vi "RunTest.vi"(8 "error in (no error)":errorcluster, 11 "Prueba05 in":refnum<class "Prueba05.lvclass">) -> (0 "error out":errorcluster, 2 "resultado":string, 3 "Prueba05 out":refnum<class "Prueba05.lvclass">)   [LabVIEW 2019, in "Prueba05.lvclass"]
uses:
  Prueba05.lvclass
  Prueba04/Control/Slide.ctl
  Prueba05.lvclass/Prueba05.ctl
  ClusterGEN.ctl
  <vilib>/Utility/miscctls.llb/LVRowAndColumnTypeDef.ctl
  <vilib>/Utility/error.llb/DialogType.ctl
  QMH/Message Queue/Enqueue Message (Single).vi
  <vilib>/Utility/error.llb/Error Cluster From Error Code.vi
  <vilib>/ErrorRing/Error Ring.xnode
  Prueba/Prueba.lvclass
  Prueba04/Prueba04.lvclass
  QMH/User Event - Stop/User Event - Stop.lvlib
  QMH/Message Queue/Message Queue.lvlib
panel:
  out "cumple_no_cumple":bool
  in  "Tab":enum32{"Page 1", "Page 2"}(tab)
  in  "generar_1":bool
  out "frecuencia":dbl
  in  "seguir":bool
  out "voltaje1":dbl format="%.1f"
  out "frecuencia1":dbl format="%.1f"
  in  "AjusteAmp":T1=50.0 caption="Ajuste de amplitud [mV]" scale=0.0..500.0
  in  "guardar":bool
  out "Pict Ring 2":u16(ring)
  out "Pict Ring":u16(ring)
  out "voltajeGuardado":dbl format="%.1f"
  in  "Tabla_A":string[][](table)
  out "voltaje2":dbl format="%.1f"
  out "frecuencia2":dbl format="%.1f"
  out "no_cumple":bool
  out "cumple":bool
  in  "generar_2":bool
  out "frecuencia2":dbl format="%.1f"
  in  "salir":bool
  # "Generación Señal de Prueba"
  # "Hz"
  # "Frecuencia"
  # "5. Ponderaciones frecuenciales y temporales a 1 KHz. IEC 61672-3: 2006 Cláusula 13"
  # "Monitoreo"
  # "Frecuencia"
  # "Hz"
  # "Voltaje"
  # "mV"
  # "Hz"
  # "mV"
  # "Cumple"
  # "No Cumple"
  # "Monitoreo"
  # "Frecuencia"
  # "Hz"
  # "Voltaje"
  # "mV"
  # "Voltaje"
  # "Frecuencia"
  # "5. Ponderaciones frecuenciales y temporales a 1 KHz. IEC 61672-3: 2006 Cláusula 13"
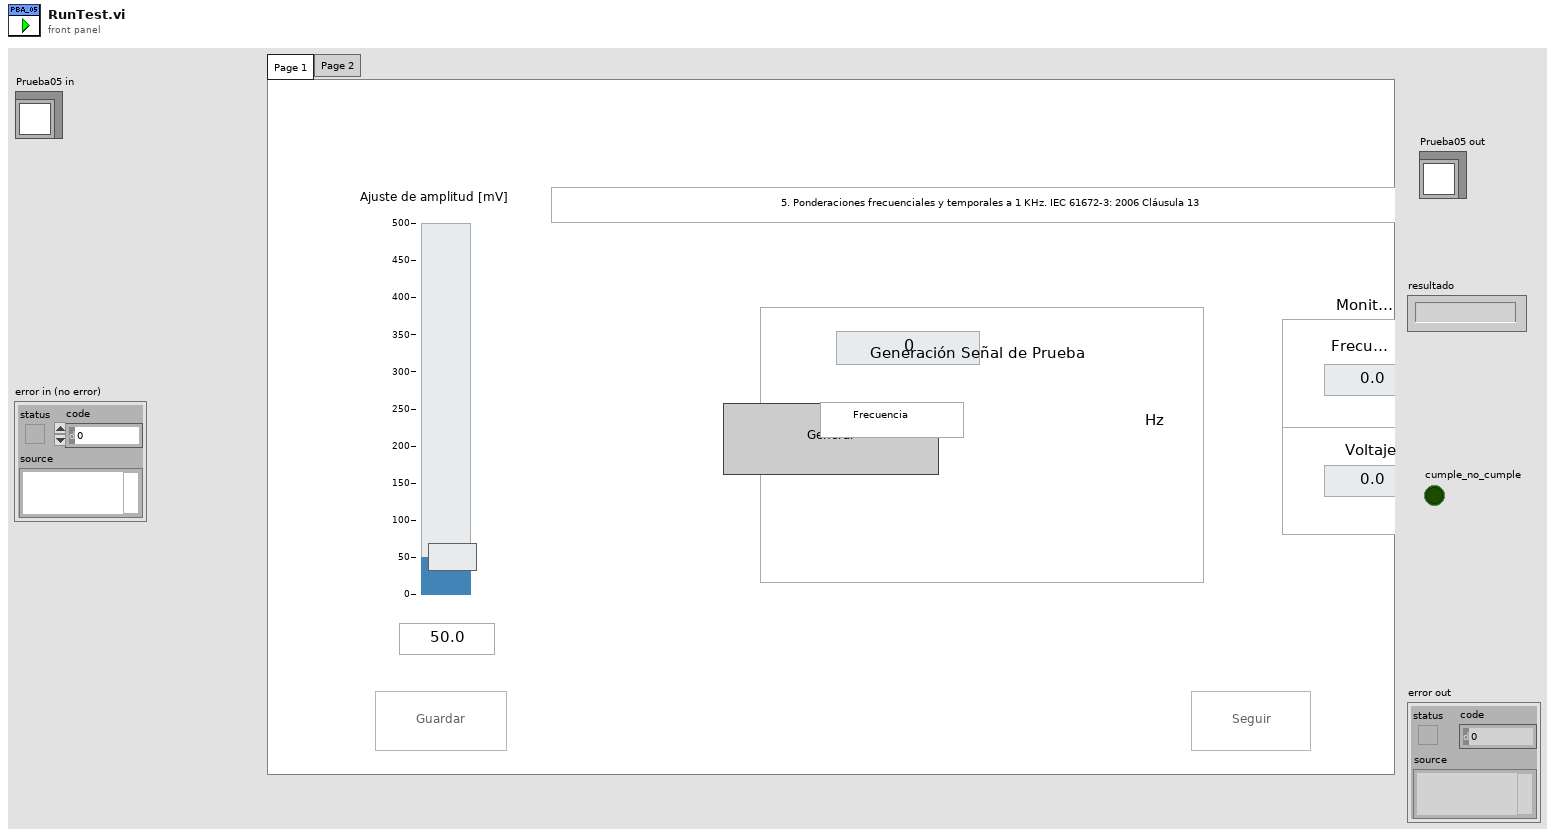
[diagram p1: front panel]
types:
  T1 = typedef "Prueba04.lvclass/Slide.ctl" = dbl
  T2 = typedef "Message Queue.lvlib/All Message Queues.ctl" = cluster{"MHL":refnum<queue>, "Inst_CNT90":refnum<queue>, "Inst_DS360":refnum<queue>, "Inst_Keithley2002":refnum<queue>, "Inst_DAQ":refnum<queue>, "BD":refnum<queue>, "Pistofono":refnum<queue>, "Nexus":refnum<queue>}
  T3 = enum8{"Enabled", "Disabled", "Disabled and Grayed Out"}
  T4 = typedef "LVRowAndColumnTypeDef.ctl" = cluster{"Row":i32, "Column":i32}
  T5 = enum32{"Page 1", "Page 2", "Page 3", "Page 4", "Page 5", "Page 6", "Page 7"}
  T6 = typedef "Prueba05.lvclass/ClusterGEN.ctl" = cluster{"frec":dbl, "amp":dbl}
  T7 = cluster{"ControlName":string, "ControlReference":refnum<vi>}[]
  T8 = typedef "DialogType.ctl" = u16
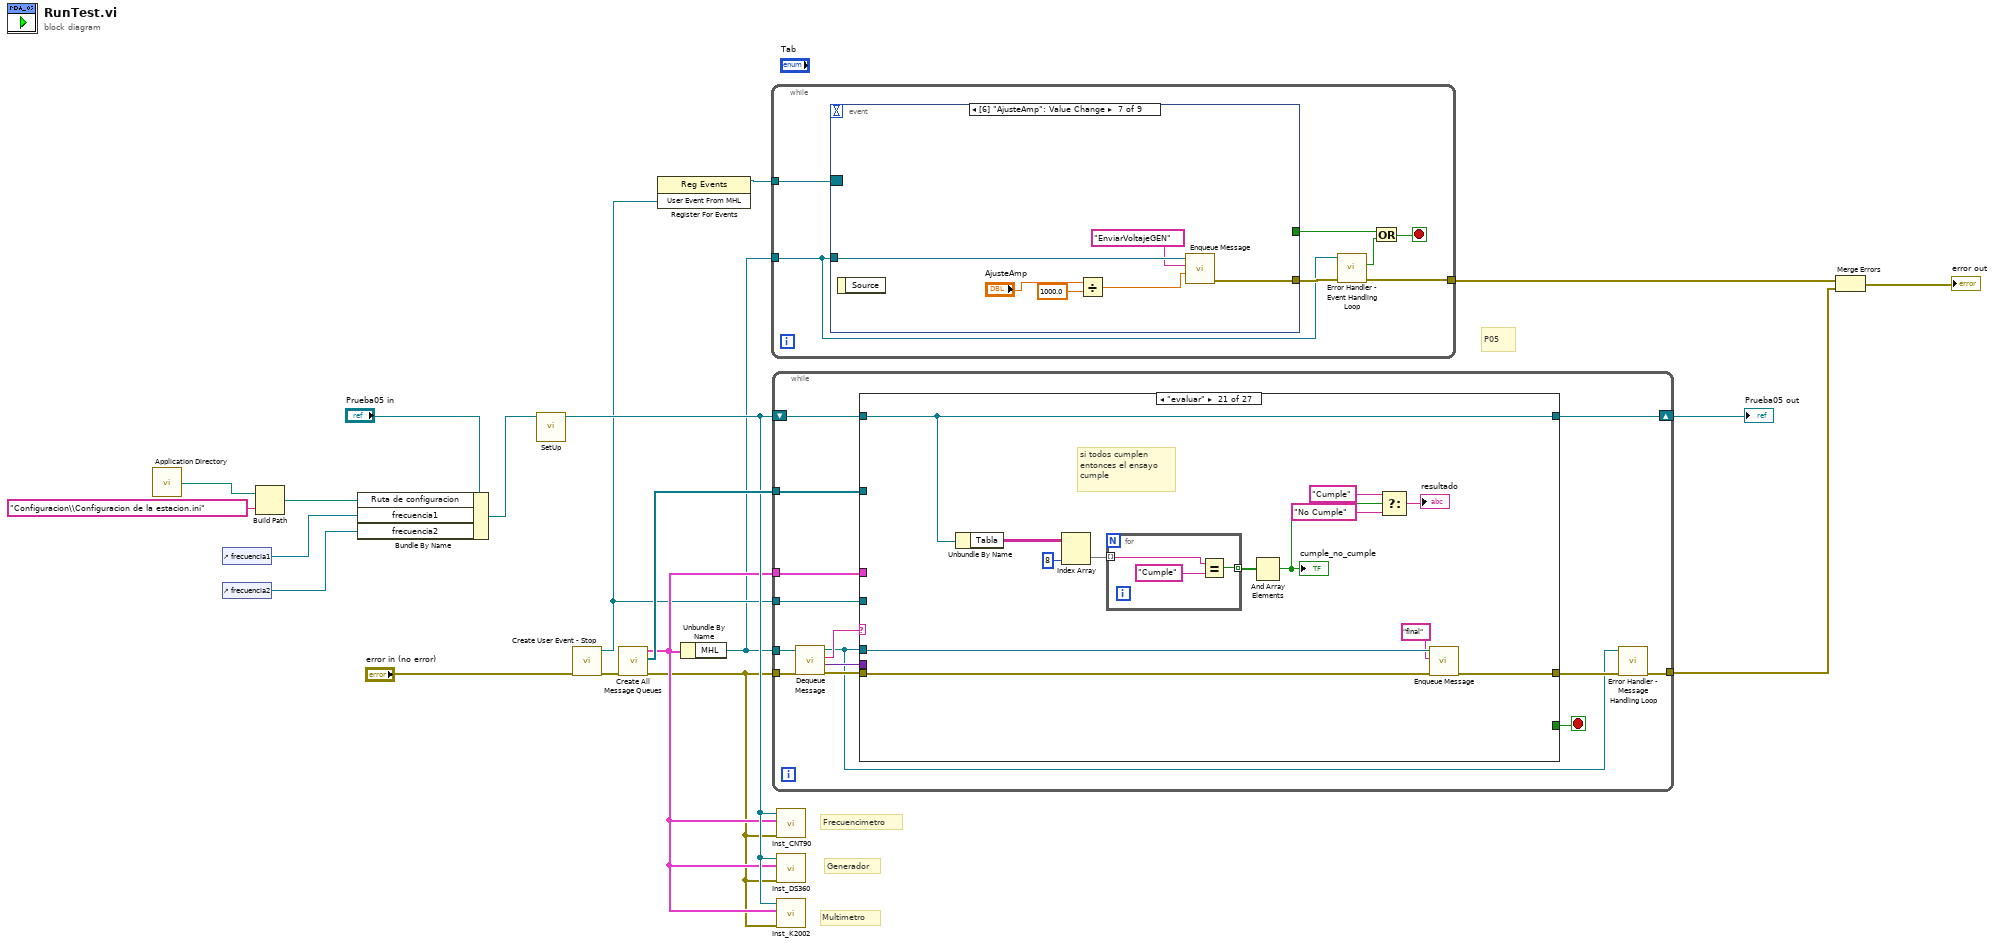
[diagram p0: block diagram]
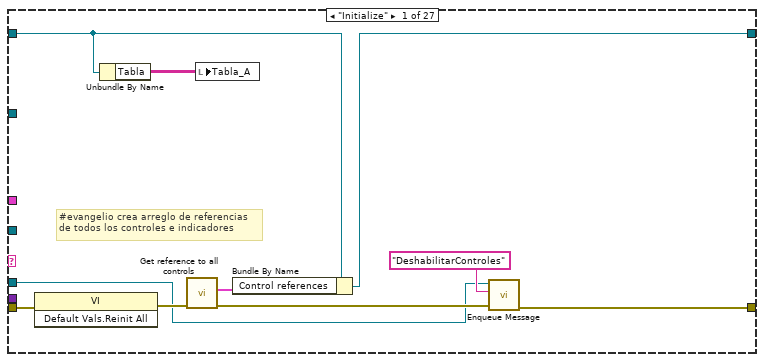
[diagram p2: hidden frame]
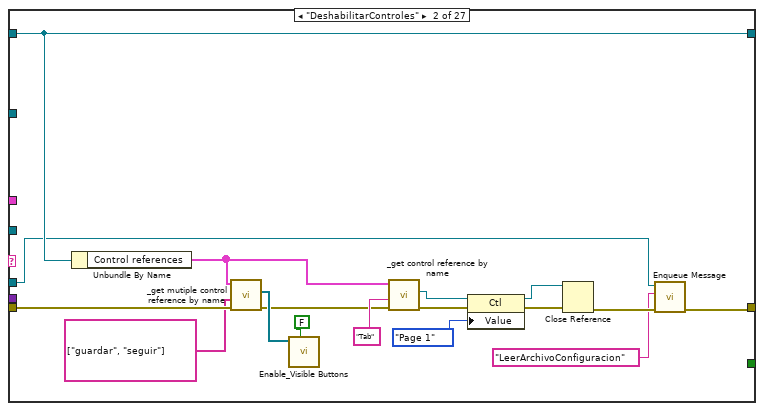
[diagram p3: hidden frame]
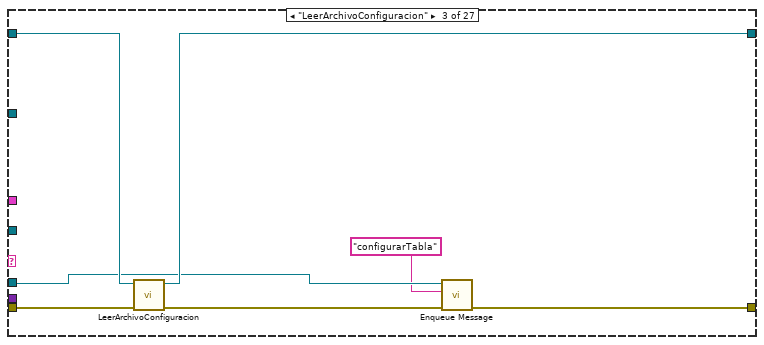
[diagram p4: hidden frame]
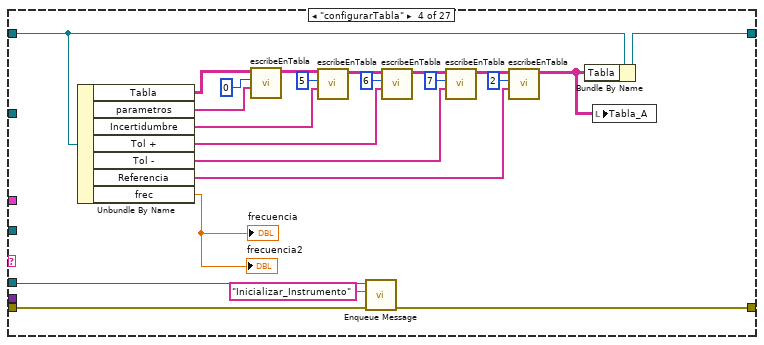
[diagram p5: hidden frame]
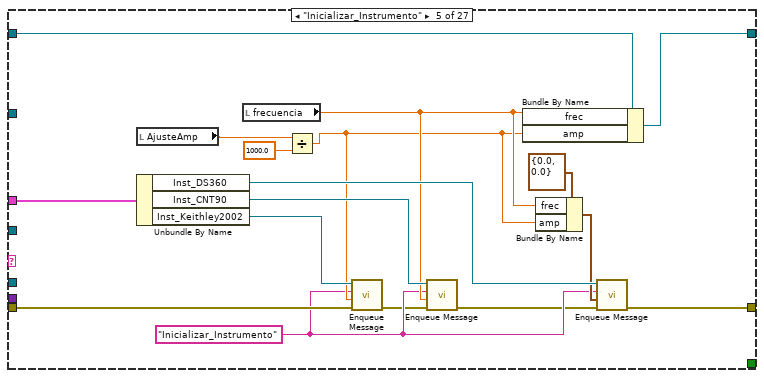
[diagram p6: hidden frame]
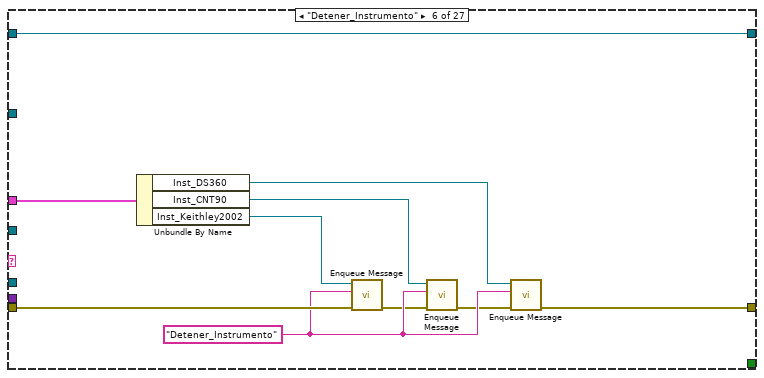
[diagram p7: hidden frame]
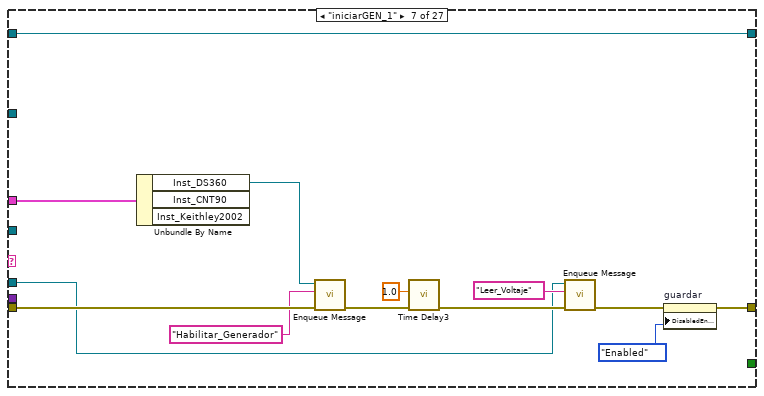
[diagram p8: hidden frame]
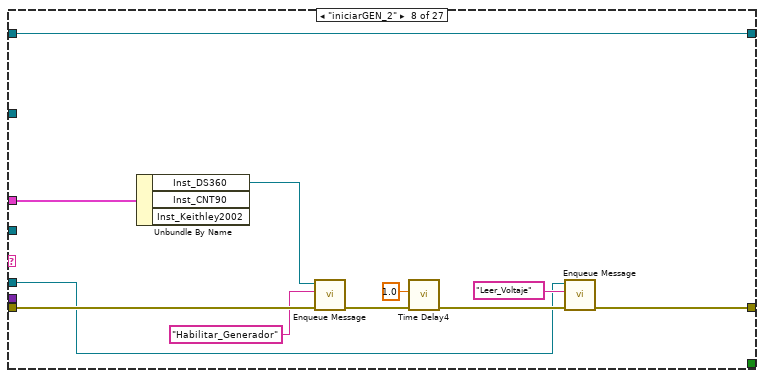
[diagram p9: hidden frame]
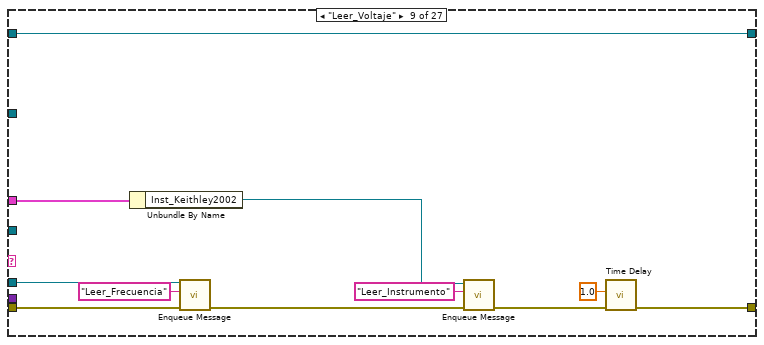
[diagram p10: hidden frame]
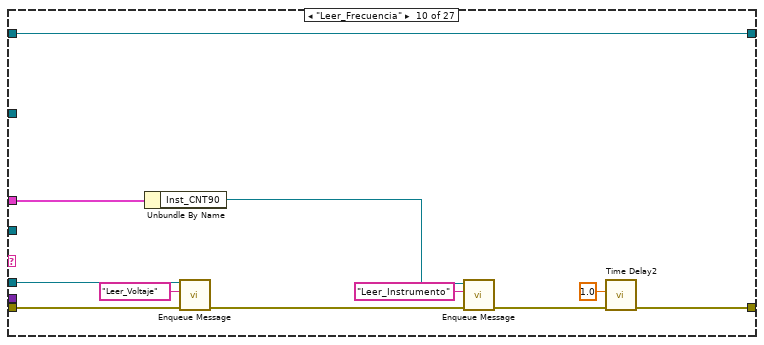
[diagram p11: hidden frame]
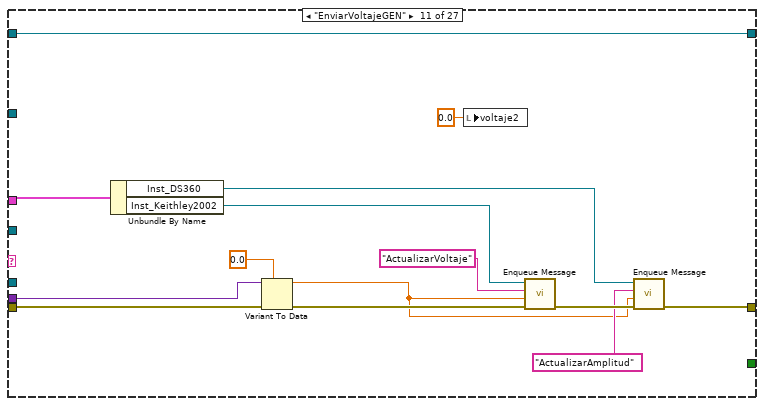
[diagram p12: hidden frame]
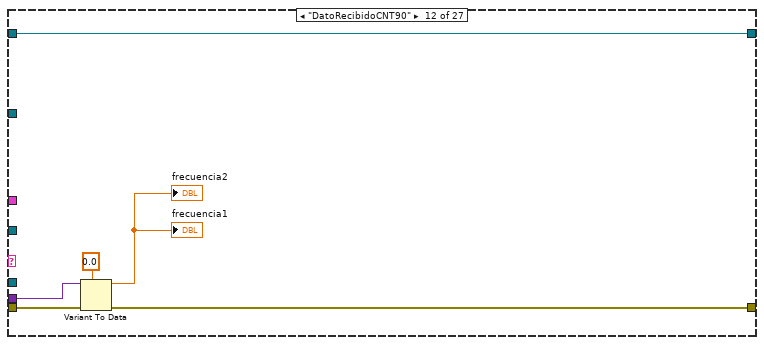
[diagram p13: hidden frame]
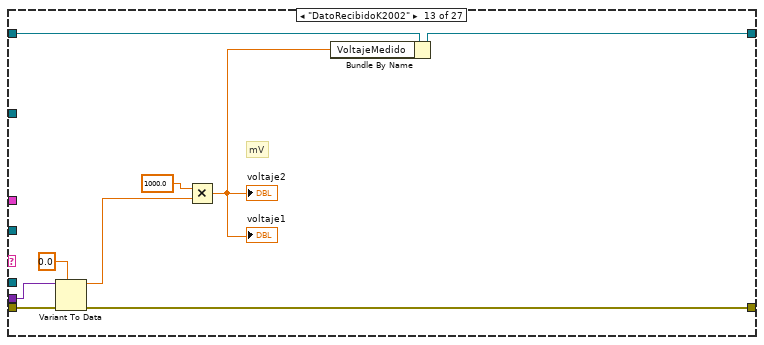
[diagram p14: hidden frame]
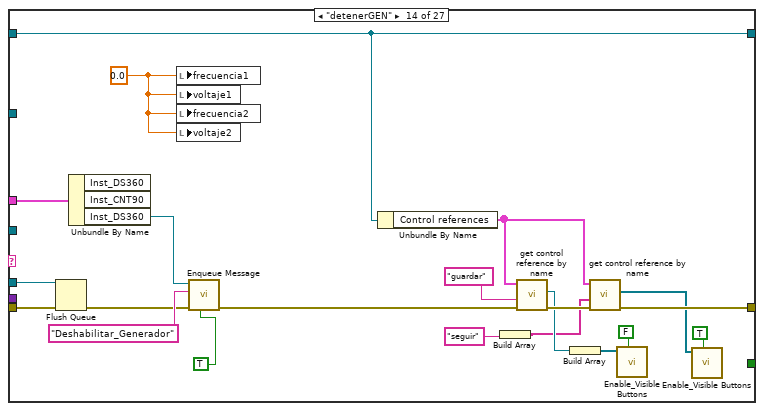
[diagram p15: hidden frame]
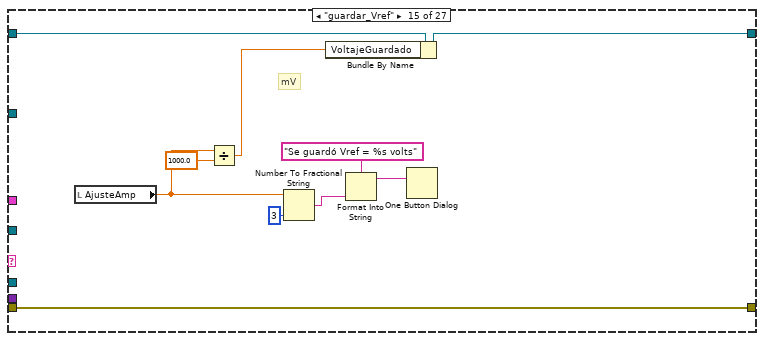
[diagram p16: hidden frame]
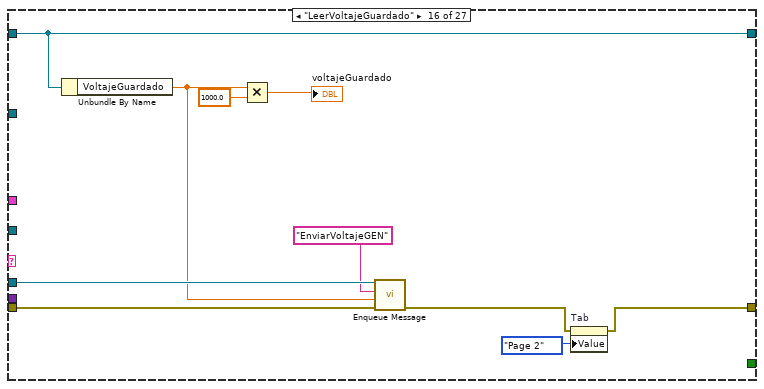
[diagram p17: hidden frame]
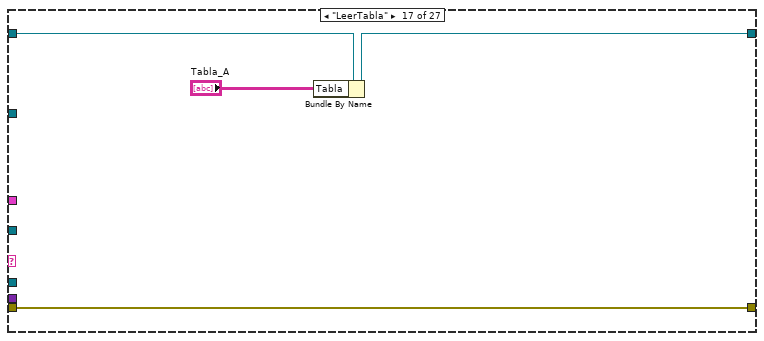
[diagram p18: hidden frame]
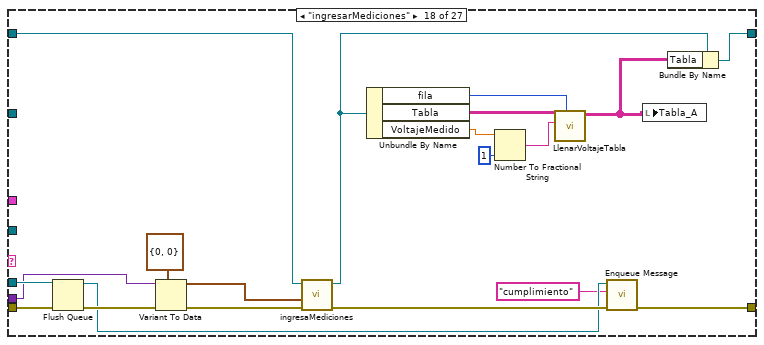
[diagram p19: hidden frame]
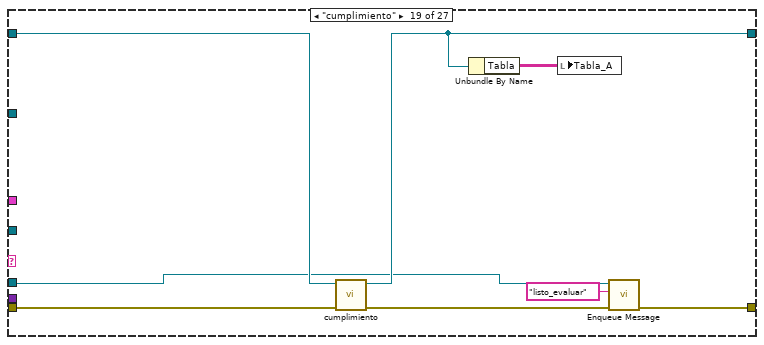
[diagram p20: hidden frame]
diagram:
  # "P05"
  # "Multimetro"
  # "Generador"
  # "Frecuencimetro"
  n1 = call <vilib>:"Application Directory.vi"() -> ("Application Directory"=w15:path)
  n2 = control-ref of="frecuencia1"() -> (w2:refnum<vi>)
  n3 = control-ref of="frecuencia2"() -> (w1:refnum<vi>)
  n4 = Build Path(base path=w15, name or relative path="Configuracion\\Configuracion de la estacion.ini") -> (appended path=w14:path)
  n5 = Bundle By Name(cluster="Prueba05 in", "Ruta de configuracion"=w14, "frecuencia1"=w2, "frecuencia2"=w1) -> (w12:refnum<class "Prueba05.lvclass">)
  n6 = call-dynamic "SetUp.vi"("Prueba05 in"=w12) -> ("Prueba05 out"=w7:refnum<class "Prueba05.lvclass">)  [unwired: 9 in, 1 out]
  n7 = call "Create User Event - Stop.vi"("error in (no error)"="error in (no error)") -> ("error out"=w11:errorcluster, "User Event From MHL"=w4:refnum<user-event>)  [unwired: 9 in]
  n8 = call "Create All Message Queues.vi"("error in (no error)"=w11) -> ("error out"=w5:errorcluster, "PL Queues Array"=w9:refnum<queue>[], "All Message Queues out"=w6:T2)  [unwired: 8 in]
  n9 = register-events(w4) -> (reference out=w8:refnum<event-registration>)  [unwired: 2 in, 1 out]
  n10 = Unbundle By Name(w6) -> ("MHL"=w3:refnum<queue>)
  n11 = while {
    tunnel: [w24] -> w20
    tunnel: w8 -> [w26]
    tunnel: w3 -> [w21]
    stop <- w27 stop-if-true
    n12 = event shown="[6] \"AjusteAmp\": Value Change" {
      selector: w26 -> [_ _ _ _ _ _ _ _ _]
      dyn-events: _ -> [_ _ _ _ _ _ _ _ _]
      timeout: _ -> [_ _ _ _ _ _ _ _ _]
      tunnel: [w32 _ w39 w44 w55 w57 w66 w67 w78] -> w25
      tunnel: w21 -> [w30 _ w41 w49 w54 w59 w65 w71 w82]
      tunnel: [_ w33 _ _ _ _ _ _ _] -> w22
      event "salir": Value Change {
        n13 = event-data() -> ()  [unwired: 1 in, 1 out]
        n14 = call-poly "Enqueue Message.vi"("Message"="Detener_Instrumento", "Message Queue"=w30) -> ("dup Message Queue"=w29:refnum<queue>)  [unwired: 8 in, 1 out]
        n15 = call-poly "Enqueue Message.vi"("Message"="Exit", "Message Queue"=w29) -> ("error out"=w32:errorcluster)  [unwired: 8 in, 1 out]
      }
      event User Event {
        n16 = event-data() -> ("User Event"=w35:string, "Event Data"=w34:variant)  [unwired: 1 in]
        n17 = case shown="\"Exit EHL\"" w35 {
          tunnel: w34 -> [_ w37]
          tunnel: [_ w36] -> w33
          frame Default {
          }
          frame "Exit EHL" {
            # "#evangelio Termina\nla ejecucion del EHL"
            n18 = Variant To Data(type=TRUE, Variant=w37) -> (data=w36:bool)  [unwired: 1 in, 1 out]
          }
        }
      }
      event Panel Close? {
        w40 = TRUE
        n19 = event-data() -> ()  [unwired: 1 in, 1 out]
        n20 = call-poly "Enqueue Message.vi"("Priority Message? (F)"=w40, "Message"="Confirmar Salida", "Message Queue"=w41) -> ("error out"=w39:errorcluster)  [unwired: 7 in, 1 out]
        n21 = event-data("Discard?"=w40) -> ()  [unwired: 1 in, 1 out]
      }
      event "generar_1": Value Change {
        n22 = event-data() -> ("NewVal"=w48:bool)  [unwired: 1 in]
        n23 = Select(t="iniciarGEN_1" ("Message"), s=w48, f="detenerGEN" ("Message")) -> (s? t:f=w45:string)
        n24 = call-poly "Enqueue Message.vi"("Priority Message? (F)"=TRUE, "Message"=w45, "Message Queue"=w49) -> ("error out"=w44:errorcluster)  [unwired: 7 in, 1 out]
      }
      event "generar_2": Value Change {
        n25 = event-data() -> ("NewVal"=w53:bool)  [unwired: 1 in]
        n26 = Select(t="iniciarGEN_2", s=w53, f="detenerGEN") -> (s? t:f=w50:string)
        n27 = call-poly "Enqueue Message.vi"("Message"=w50, "Message Queue"=w54) -> ("error out"=w55:errorcluster)  [unwired: 8 in, 1 out]
      }
      event "seguir": Value Change {
        n28 = event-data() -> ()  [unwired: 1 in, 1 out]
        n29 = call-poly "Enqueue Message.vi"("Message"="LeerVoltajeGuardado", "Message Queue"=w59) -> ("error out"=w58:errorcluster)  [unwired: 8 in, 1 out]
        n30 = property on="Tab" class="TabCtl (strict)"(error in=w58, "Value"=enum32{"Page 1", "Page 2"}."Page 2" ("Tab")) -> (error out=w57:errorcluster)  [unwired: 1 in, 1 out]
      }
      event Value Change {
        n31 = event-data() -> ()  [unwired: 1 in, 1 out]
        n32 = Divide(x="AjusteAmp", y=T1 1000.0) -> (x/y=w61:T1)
        n33 = call-poly "Enqueue Message.vi"("Message Data"=w61, "Message"="EnviarVoltajeGEN", "Message Queue"=w65) -> ("error out"=w66:errorcluster)  [unwired: 7 in, 1 out]
      }
      event "guardar": Value Change {
        n34 = event-data() -> ()  [unwired: 1 in, 1 out]
        n35 = call-poly "Enqueue Message.vi"("Message"="guardar_Vref", "Message Queue"=w71) -> ("error out"=w68:errorcluster)  [unwired: 8 in, 1 out]
        n36 = property on="seguir" class="Bool"(error in=w68, "DisabledEnum"=T3."Enabled" ("Disabled")) -> (error out=w67:errorcluster)  [unwired: 1 in, 1 out]
      }
      event "Tabla_A": Value Change {
        n37 = event-data() -> ("CtlRef"=w81:refnum<vi>)  [unwired: 1 in]
        n38 = Flush Queue(queue=w82) -> (queue out=w74:refnum<queue>, error out=w72:errorcluster)  [unwired: 1 in, 1 out]
        n39 = property class="Tbl (strict)"(reference=w81, error in=w72) -> (error out=w73:errorcluster, "Selection Start"=w77:T4)  [unwired: 1 out]
        n40 = call-poly "Enqueue Message.vi"("error in (no error)"=w73, "Message"="LeerTabla", "Message Queue"=w74) -> ("error out"=w79:errorcluster, "dup Message Queue"=w80:refnum<queue>)  [unwired: 7 in]
        n41 = call-poly "Enqueue Message.vi"("error in (no error)"=w79, "Message Data"=w77, "Message"="ingresarMediciones", "Message Queue"=w80) -> ("error out"=w78:errorcluster)  [unwired: 6 in, 1 out]
      }
    }
    n42 = call "Error Handler - Event Handling Loop.vi"("error in (no error)"=w25, "Message Queue"=w21) -> ("dup error in"=w24:errorcluster, "Error?"=w23:bool)  [unwired: 7 in, 1 out]
    n43 = Or(x=w22, y=w23) -> (x .or. y?=w27:bool)
  }
  n44 = while {
    tunnel: [w87] -> w19
    shift-right: [w95] -> w17
    shift-left: w7 -> [w96]
    tunnel: w5 -> [w94]
    tunnel: w3 -> [w92]
    tunnel: w6 -> [w86]
    tunnel: w9 -> [w85]
    tunnel: w4 -> [w84]
    stop <- w83 stop-if-true
    n45 = call "Dequeue Message.vi"("error in (no error)"=w94, "Message Queue"=w92) -> ("error out"=w93:errorcluster, "Message Data"=w90:variant, "Message"=w91:string, "dup Message Queue"=w88:refnum<queue>)  [unwired: 6 in]
    n46 = case shown="\"evaluar\"" w91 {
      selector: w91 -> [_ _ _ _ _ _ _ _ _ _ _ _ _ _ _ _ _ _ _ _ _ _ w374 _ _ w415 w425]
      tunnel: w93 -> [w101 w118 w130 w153 w170 w180 w193 w204 w215 w226 w229 w246 w255 w271 w285 w294 w299 w319 w327 w336 w360 w370 w379 w390 w407 _ _]
      tunnel: [w106 w109 w126 w133 w154 w171 w187 w194 w206 w217 w228 w243 w253 w267 w285 w293 w299 w317 w325 w332 w356 w366 w378 w388 w405 w414 w424] -> w89
      tunnel: w88 -> [w97 w108 w125 w132 _ _ w182 w195 w212 w223 _ _ _ w270 _ w290 _ w310 w321 w329 w353 w365 w380 w389 w406 _ _]
      tunnel: w96 -> [w100 w117 w128 w137 w169 w179 w192 w203 w214 w225 w240 w245 w254 w258 w280 w292 w298 w313 w324 w331 w355 w367 w371 w395 w413 w416 w426]
      tunnel: [w99 w117 w127 w135 w168 w179 w192 w203 w214 w225 w240 w245 w248 w258 w279 w292 w297 w300 w323 w331 w355 w367 w371 w395 w413 w416 w426] -> w95
      tunnel: w90 -> [_ _ _ _ _ _ _ _ _ _ w230 w244 w252 _ _ _ _ w308 _ _ _ _ _ _ w404 _ _]
      tunnel: w86 -> [_ _ _ _ w164 w178 w191 w202 w209 w220 w231 _ _ w269 _ _ _ _ _ _ _ _ _ _ _ _ _]
      tunnel: w85 -> [_ _ _ _ _ _ _ _ _ _ _ _ _ _ _ _ _ _ _ _ _ _ w376 _ _ _ _]
      tunnel: w84 -> [_ _ _ _ _ _ _ _ _ _ _ _ _ _ _ _ _ _ _ _ _ _ w377 _ _ _ _]
      tunnel: [_ _ _ _ _ _ _ _ _ _ _ _ _ _ _ _ _ _ _ _ _ _ w375 _ _ _ _] -> w83
      frame "Initialize" {
        # "#evangelio crea arreglo de referencias\nde todos los controles e indicadores"
        n47 = invoke class="VI" method="Default Vals.Reinit All"(error in=w101) -> (error out=w103:errorcluster)  [unwired: 2 in, 2 out]
        n48 = Unbundle By Name(w100) -> ("Tabla"=w105:string[][])
        n49 = call "Get reference to all controls.vi"("error in (no error)"=w103) -> ("error out"=w98:errorcluster, "Control references"=w102:T7)  [unwired: 5 in]
        n50 = local write "Tabla_A"(w105) -> ()
        n51 = Bundle By Name(cluster=w100, "Control references"=w102) -> (w99:refnum<class "Prueba05.lvclass">)
        n52 = call-poly "Enqueue Message.vi"("error in (no error)"=w98, "Message"="DeshabilitarControles", "Message Queue"=w97) -> ("error out"=w106:errorcluster)  [unwired: 7 in, 1 out]
      }
      frame "DeshabilitarControles" {
        n53 = Unbundle By Name(w117) -> ("Control references"=w119:T7)
        n54 = call "_get mutiple control reference by name.vi"("error in (no error)"=w118, "Control names"=string[] ["guardar", "seguir"], "Control references"=w119) -> ("error out"=w114:errorcluster, "References"=w115:refnum<vi>[])  [unwired: 3 in]
        n55 = call "Enable_Visible Buttons.vi"("Enable? (T)"=FALSE, "Controls Ref Array"=w115) -> ()  [unwired: 10 in]
        n56 = call "_get control reference by name.vi"("error in (no error)"=w114, "Control name"="Tab" ("Message"), "Control references"=w119) -> ("error out"=w123:errorcluster, "Ctl Refnum"=w121:refnum<vi>)  [unwired: 3 in]
        n57 = property class="Ctl"(reference=w121, error in=w123, "Value"=T5."Page 1" ("Tab_Prueba04")) -> (reference out=w110:refnum<vi>, error out=w112:errorcluster)
        n58 = Close Reference(reference=w110, error in (no error)=w112) -> (error out=w111:errorcluster)
        n59 = call-poly "Enqueue Message.vi"("error in (no error)"=w111, "Message"="LeerArchivoConfiguracion", "Message Queue"=w108) -> ("error out"=w109:errorcluster)  [unwired: 7 in, 1 out]
      }
      frame "LeerArchivoConfiguracion" {
        n60 = call "LeerArchivoConfiguracion.vi"("error in"=w130, "Prueba05 in"=w128) -> ("error out"=w129:errorcluster, "Prueba05 out"=w127:refnum<class "Prueba05.lvclass">)  [unwired: 8 in]
        n61 = call-poly "Enqueue Message.vi"("error in (no error)"=w129, "Message"="configurarTabla", "Message Queue"=w125) -> ("error out"=w126:errorcluster)  [unwired: 7 in, 1 out]
      }
      frame "configurarTabla" {
        n62 = Unbundle By Name(w137) -> ("Tabla"=w136:string[][], "parametros"=w151:string[], "Incertidumbre"=w144:string[], "Tol +"=w143:string[], "Tol -"=w142:string[], "Referencia"=w139:string[], "frec"=→"frecuencia" →"frecuencia2":dbl)
        n63 = call "escribeEnTabla.vi"("parametros"=w151, "col"=0, "tabla in"=w136) -> ("tabla out"=w145:string[][])  [unwired: 8 in]
        n64 = call "escribeEnTabla.vi"("parametros"=w144, "col"=5, "tabla in"=w145) -> ("tabla out"=w150:string[][])  [unwired: 8 in]
        n65 = call-poly "Enqueue Message.vi"("error in (no error)"=w153, "Message"="Inicializar_Instrumento", "Message Queue"=w132) -> ("error out"=w133:errorcluster)  [unwired: 7 in, 1 out]
        n66 = call "escribeEnTabla.vi"("parametros"=w143, "col"=6, "tabla in"=w150) -> ("tabla out"=w149:string[][])  [unwired: 8 in]
        n67 = call "escribeEnTabla.vi"("parametros"=w142, "col"=7, "tabla in"=w149) -> ("tabla out"=w140:string[][])  [unwired: 8 in]
        n68 = call "escribeEnTabla.vi"("parametros"=w139, "col"=2, "tabla in"=w140) -> ("tabla out"=w134:string[][])  [unwired: 8 in]
        n69 = Bundle By Name(cluster=w137, "Tabla"=w134) -> (w135:refnum<class "Prueba05.lvclass">)
        n70 = local write "Tabla_A"(w134) -> ()
      }
      frame "Inicializar_Instrumento" {
        w157 = "Inicializar_Instrumento" ("Message")
        n71 = local read "AjusteAmp"() -> (w166:T1)
        n72 = Unbundle By Name(w164) -> ("Inst_DS360"=w163:refnum<queue>, "Inst_CNT90"=w162:refnum<queue>, "Inst_Keithley2002"=w161:refnum<queue>)
        n73 = local read "frecuencia"() -> (w159:dbl)
        n74 = Divide(x=w166, y=T1 1000.0) -> (x/y=w158:T1)
        n75 = call-poly "Enqueue Message.vi"("error in (no error)"=w170, "Message Data"=w158, "Message"=w157, "Message Queue"=w161) -> ("error out"=w156:errorcluster)  [unwired: 6 in, 1 out]
        n76 = call-poly "Enqueue Message.vi"("error in (no error)"=w156, "Message Data"=w159, "Message"=w157, "Message Queue"=w162) -> ("error out"=w155:errorcluster)  [unwired: 6 in, 1 out]
        n77 = Bundle By Name(cluster=w169, "frec"=w159, "amp"=w158) -> (w168:refnum<class "Prueba05.lvclass">)
        n78 = Bundle By Name(cluster=T6 {"frec"=0.0, "amp"=0.0}, "frec"=w159, "amp"=w158) -> (w160:T6)
        n79 = call-poly "Enqueue Message.vi"("error in (no error)"=w155, "Message Data"=w160, "Message"=w157, "Message Queue"=w163) -> ("error out"=w154:errorcluster)  [unwired: 6 in, 1 out]
      }
      frame "Detener_Instrumento" {
        w174 = "Detener_Instrumento" ("Message")
        n80 = Unbundle By Name(w178) -> ("Inst_DS360"=w177:refnum<queue>, "Inst_CNT90"=w176:refnum<queue>, "Inst_Keithley2002"=w175:refnum<queue>)
        n81 = call-poly "Enqueue Message.vi"("error in (no error)"=w180, "Message"=w174, "Message Queue"=w175) -> ("error out"=w173:errorcluster)  [unwired: 7 in, 1 out]
        n82 = call-poly "Enqueue Message.vi"("error in (no error)"=w173, "Message"=w174, "Message Queue"=w176) -> ("error out"=w172:errorcluster)  [unwired: 7 in, 1 out]
        n83 = call-poly "Enqueue Message.vi"("error in (no error)"=w172, "Message"=w174, "Message Queue"=w177) -> ("error out"=w171:errorcluster)  [unwired: 7 in, 1 out]
      }
      frame "iniciarGEN_1" {
        n84 = Unbundle By Name(w191) -> ("Inst_DS360"=w190:refnum<queue>)  [unwired: 2 out]
        n85 = call-poly "Enqueue Message.vi"("error in (no error)"=w193, "Message"="Habilitar_Generador", "Message Queue"=w190) -> ("error out"=w185:errorcluster)  [unwired: 7 in, 1 out]
        n86 = call "Time Delay3"("error in (no error)"=w185, "Delay Time (s)"=1.0) -> ("error out"=w184:errorcluster)  [unwired: 9 in]
        n87 = call-poly "Enqueue Message.vi"("error in (no error)"=w184, "Message"="Leer_Voltaje", "Message Queue"=w182) -> ("error out"=w181:errorcluster)  [unwired: 7 in, 1 out]
        n88 = property on="guardar" class="Bool"(error in=w181, "DisabledEnum"=T3."Enabled" ("Disabled")) -> (error out=w187:errorcluster)  [unwired: 1 in, 1 out]
      }
      frame "iniciarGEN_2" {
        n89 = Unbundle By Name(w202) -> ("Inst_DS360"=w201:refnum<queue>)  [unwired: 2 out]
        n90 = call-poly "Enqueue Message.vi"("error in (no error)"=w204, "Message"="Habilitar_Generador", "Message Queue"=w201) -> ("error out"=w198:errorcluster)  [unwired: 7 in, 1 out]
        n91 = call "Time Delay4"("error in (no error)"=w198, "Delay Time (s)"=1.0) -> ("error out"=w197:errorcluster)  [unwired: 9 in]
        n92 = call-poly "Enqueue Message.vi"("error in (no error)"=w197, "Message"="Leer_Voltaje", "Message Queue"=w195) -> ("error out"=w194:errorcluster)  [unwired: 7 in, 1 out]
      }
      frame "Leer_Voltaje" {
        n93 = Unbundle By Name(w209) -> ("Inst_Keithley2002"=w208:refnum<queue>)
        n94 = call-poly "Enqueue Message.vi"("error in (no error)"=w215, "Message"="Leer_Frecuencia", "Message Queue"=w212) -> ("error out"=w213:errorcluster)  [unwired: 7 in, 1 out]
        n95 = call-poly "Enqueue Message.vi"("error in (no error)"=w213, "Message"="Leer_Instrumento", "Message Queue"=w208) -> ("error out"=w210:errorcluster)  [unwired: 7 in, 1 out]
        n96 = call "Time Delay"("error in (no error)"=w210, "Delay Time (s)"=1.0) -> ("error out"=w206:errorcluster)  [unwired: 9 in]
      }
      frame "Leer_Frecuencia" {
        n97 = Unbundle By Name(w220) -> ("Inst_CNT90"=w219:refnum<queue>)
        n98 = call-poly "Enqueue Message.vi"("error in (no error)"=w226, "Message"="Leer_Voltaje", "Message Queue"=w223) -> ("error out"=w224:errorcluster)  [unwired: 7 in, 1 out]
        n99 = call-poly "Enqueue Message.vi"("error in (no error)"=w224, "Message"="Leer_Instrumento", "Message Queue"=w219) -> ("error out"=w221:errorcluster)  [unwired: 7 in, 1 out]
        n100 = call "Time Delay2"("error in (no error)"=w221, "Delay Time (s)"=1.0) -> ("error out"=w217:errorcluster)  [unwired: 9 in]
      }
      frame "EnviarVoltajeGEN" {
        n101 = Unbundle By Name(w231) -> ("Inst_DS360"=w234:refnum<queue>, "Inst_Keithley2002"=w239:refnum<queue>)
        n102 = Variant To Data(error in=w229, type=0.0, Variant=w230) -> (data=w232:dbl, error out=w237:errorcluster)
        n103 = local write "voltaje2"(0.0 ("voltaje2")) -> ()
        n104 = call-poly "Enqueue Message.vi"("error in (no error)"=w237, "Message Data"=w232, "Message"="ActualizarVoltaje", "Message Queue"=w239) -> ("error out"=w235:errorcluster)  [unwired: 6 in, 1 out]
        n105 = call-poly "Enqueue Message.vi"("error in (no error)"=w235, "Message Data"=w232, "Message"="ActualizarAmplitud", "Message Queue"=w234) -> ("error out"=w228:errorcluster)  [unwired: 6 in, 1 out]
      }
      frame "DatoRecibidoCNT90" {
        n106 = Variant To Data(error in=w246, type=0.0, Variant=w244) -> (data=→"frecuencia2" →"frecuencia1":dbl, error out=w243:errorcluster)
      }
      frame "DatoRecibidoK2002" {
        # "mV"
        n107 = Variant To Data(error in=w255, type=0.0 ("x"), Variant=w252) -> (data=w249:dbl, error out=w253:errorcluster)
        n108 = Multiply(x=1000.0, y=w249) -> (x*y=w247:dbl)
        "voltaje2" <- w247
        "voltaje1" <- w247
        n109 = Bundle By Name(cluster=w254, "VoltajeMedido"=w247) -> (w248:refnum<class "Prueba05.lvclass">)
      }
      frame "detenerGEN" {
        w275 = 0.0 ("frecuencia1")
        n110 = Flush Queue(queue=w270, error in (no error)=w271) -> (error out=w257:errorcluster)  [unwired: 2 out]
        n111 = Unbundle By Name(w269) -> ("Inst_DS360"=w274:refnum<queue>)  [unwired: 2 out]
        n112 = local write "frecuencia1"(w275) -> ()
        n113 = local write "voltaje1"(w275) -> ()
        n114 = local write "frecuencia2"(w275) -> ()
        n115 = local write "voltaje2"(w275) -> ()
        n116 = call-poly "Enqueue Message.vi"("Priority Message? (F)"=TRUE, "error in (no error)"=w257, "Message"="Deshabilitar_Generador", "Message Queue"=w274) -> ("error out"=w256:errorcluster)  [unwired: 6 in, 1 out]
        n117 = Unbundle By Name(w258) -> ("Control references"=w262:T7)
        n118 = Build Array("seguir" ("String")) -> (w259:string[])
        n119 = call-poly "get control reference by name.vi"("error in (no error)"=w256, "Control name"="guardar" ("String"), "Control references"=w262) -> ("error out"=w267:errorcluster, "Ctl Refnum"=w265:refnum<vi>)  [unwired: 3 in]
        n120 = Build Array(w265) -> (w264:refnum<vi>[])
        n121 = call-poly "get control reference by name.vi"("Control names"=w259, "Control references"=w262) -> ("References"=w261:refnum<vi>[])  [unwired: 4 in, 1 out]
        n122 = call "Enable_Visible Buttons.vi"("Enable? (T)"=FALSE, "Controls Ref Array"=w264) -> ()  [unwired: 10 in]
        n123 = call "Enable_Visible Buttons.vi"("Enable? (T)"=TRUE, "Controls Ref Array"=w261) -> ()  [unwired: 10 in]
      }
      frame "guardar_Vref" {
        # "mV"
        n124 = local read "AjusteAmp"() -> (w278:T1)
        n125 = Divide(x=w278, y=T1 1000.0) -> (x/y=w276:T1)
        n126 = Number To Fractional String(number=w278, precision (6)=i16 3) -> (F-format string=w281:string)  [unwired: 2 in]
        n127 = Bundle By Name(cluster=w280, "VoltajeGuardado"=w276) -> (w279:refnum<class "Prueba05.lvclass">)
        n128 = Format Into String(format string="Se guardó Vref = %s volts", w281) -> (resulting string=w284:string)  [unwired: 2 in, 1 out]
        n129 = One Button Dialog(message=w284) -> ()  [unwired: 1 in, 1 out]
      }
      frame "LeerVoltajeGuardado" {
        n130 = Unbundle By Name(w292) -> ("VoltajeGuardado"=w286:dbl)
        n131 = Multiply(x=w286, y=1000.0) -> (x*y=→"voltajeGuardado":dbl)
        n132 = call-poly "Enqueue Message.vi"("error in (no error)"=w294, "Message Data"=w286, "Message"="EnviarVoltajeGEN", "Message Queue"=w290) -> ("error out"=w291:errorcluster)  [unwired: 6 in, 1 out]
        n133 = property on="Tab" class="TabCtl (strict)"(error in=w291, "Value"=enum32{"Page 1", "Page 2"}."Page 2" ("Tab")) -> (error out=w293:errorcluster)  [unwired: 1 in, 1 out]
      }
      frame "LeerTabla" {
        n134 = Bundle By Name(cluster=w298, "Tabla"="Tabla_A") -> (w297:refnum<class "Prueba05.lvclass">)
      }
      frame "ingresarMediciones" {
        n135 = Flush Queue(queue=w310, error in (no error)=w319) -> (queue out=w314:refnum<queue>, error out=w315:errorcluster)  [unwired: 1 out]
        n136 = Variant To Data(error in=w315, type=T4 {"Row"=0, "Column"=0} ("Selection Start"), Variant=w308) -> (data=w311:T4, error out=w316:errorcluster)
        n137 = call "ingresaMediciones.vi"("error in (no error)"=w316, "Selection Start"=w311, "Prueba05 in"=w313) -> ("error out"=w318:errorcluster, "Prueba05 out"=w301:refnum<class "Prueba05.lvclass">)  [unwired: 7 in]
        n138 = Unbundle By Name(w301) -> ("fila"=w303:i32, "Tabla"=w306:string[][], "VoltajeMedido"=w307:dbl)
        n139 = Number To Fractional String(number=w307, precision (6)=i16 1) -> (F-format string=w305:string)  [unwired: 2 in]
        n140 = call "LlenarVoltajeTabla.vi"("fila"=w303, "Dato"=w305, "Tabla in"=w306) -> ("Tabla out"=w304:string[][])  [unwired: 8 in]
        n141 = call-poly "Enqueue Message.vi"("error in (no error)"=w318, "Message"="cumplimiento", "Message Queue"=w314) -> ("error out"=w317:errorcluster)  [unwired: 7 in, 1 out]
        n142 = local write "Tabla_A"(w304) -> ()
        n143 = Bundle By Name(cluster=w301, "Tabla"=w304) -> (w300:refnum<class "Prueba05.lvclass">)
      }
      frame "cumplimiento" {
        n144 = call "cumplimiento.vi"("error in (no error)"=w327, "Prueba04 in"=w324) -> ("error out"=w326:errorcluster, "Prueba04 out"=w323:refnum<class "Prueba05.lvclass">)  [unwired: 8 in]
        n145 = Unbundle By Name(w323) -> ("Tabla"=w322:string[][])
        n146 = local write "Tabla_A"(w322) -> ()
        n147 = call-poly "Enqueue Message.vi"("error in (no error)"=w326, "Message"="listo_evaluar", "Message Queue"=w321) -> ("error out"=w325:errorcluster)  [unwired: 7 in, 1 out]
      }
      frame "listo_evaluar" {
        n148 = Unbundle By Name(w331) -> ("Tabla"=w330:string[][])
        n149 = Index Array(array=w330, index (col)=8 ("disabled index (col)")) -> (element=w334:string[])  [unwired: 1 in]
        n150 = for {
          tunnel: [w347] -> w333 mode=indexing
          tunnel: w334 -> [w345] mode=indexing
          n151 = Not Equal?(x=w345, y="--") -> (x != y?=w347:bool)
        }
        n152 = And Array Elements(Boolean array=w333) -> (logical AND=w328:bool)
        n153 = case shown="True" w328 {
          tunnel: w336 -> [w340 w344]
          tunnel: [w339 w343] -> w332
          tunnel: w329 -> [w338 w342]
          frame False {
            n154 = call-poly "Enqueue Message.vi"("error in (no error)"=w340, "Message"="Leer_Voltaje", "Message Queue"=w338) -> ("error out"=w339:errorcluster)  [unwired: 7 in, 1 out]
          }
          frame True {
            n155 = call-poly "Enqueue Message.vi"("error in (no error)"=w344, "Message"="evaluar", "Message Queue"=w342) -> ("error out"=w343:errorcluster)  [unwired: 7 in, 1 out]
          }
        }
      }
      frame "evaluar" {
        # "si todos cumplen\nentonces el ensayo\ncumple"
        n156 = Unbundle By Name(w355) -> ("Tabla"=w354:string[][])
        n157 = Index Array(array=w354, index (col)=8 ("disabled index (col)")) -> (element=w358:string[])  [unwired: 1 in]
        n158 = for {
          tunnel: [w363] -> w359 mode=indexing
          tunnel: w358 -> [w361] mode=indexing
          n159 = Equal?(x=w361, y="Cumple") -> (x = y?=w363:bool)
        }
        n160 = And Array Elements(Boolean array=w359) -> (logical AND=w351:bool)
        "cumple_no_cumple" <- w351
        n161 = Select(t="Cumple" ("y"), s=w351, f="No Cumple" ("y")) -> (s? t:f=→"resultado":string)
        n162 = call-poly "Enqueue Message.vi"("error in (no error)"=w360, "Message"="final", "Message Queue"=w353) -> ("error out"=w356:errorcluster)  [unwired: 7 in, 1 out]
      }
      frame "final" {
        n163 = local read "cumple_no_cumple"() -> (w368:bool)
        "cumple" <- w368
        n164 = call-poly "Enqueue Message.vi"("error in (no error)"=w370, "Message"="Leer_Voltaje", "Message Queue"=w365) -> ("error out"=w366:errorcluster)  [unwired: 7 in, 1 out]
        n165 = Not(x=w368) -> (.not. x?=→"no_cumple":bool)
      }
      frame "Exit" {
        w375 = TRUE
        # "#evangelio Manda a cerrar el EHL"
        # "#evangelio Manda a cerrar todos los Loops"
        n166 = Release Queue(queue=w380, error in (no error)=w379) -> (error out=w383:errorcluster)  [unwired: 1 in, 2 out]
        n167 = Unbundle By Name(w371) -> ("Control references"=w384:T7)
        n168 = for {
          tunnel: w376 -> [w387] mode=indexing
          tunnel: w374 -> [w386]
          tunnel: TRUE -> [w385]
          n169 = call-poly "Enqueue Message.vi"("Priority Message? (F)"=w385, "Message"=w386, "Message Queue"=w387) -> ()  [unwired: 7 in, 2 out]
        }
        n170 = call "Close All Ref.vi"("error in (no error)"=w383, "Control references"=w384) -> ("error out"=w373:errorcluster)  [unwired: 9 in]
        n171 = call-dynamic "CleanUp.vi"("error in (no error)"=w373, "Prueba05 in"=w371) -> ("error out"=w372:errorcluster)  [unwired: 8 in, 1 out]
        n172 = call "Fire User Event - Stop.vi"("error in (no error)"=w372, "Event Data"=w375, "User Event"="Exit EHL", "User Event in"=w377) -> ("error out"=w378:errorcluster)  [unwired: 7 in]
      }
      frame "Confirmar Salida" {
        n173 = Two Button Dialog(message="¿Quieres cerrar la aplicación?", 1:"No" ("T button name (\"OK\")"), 2:"Si" ("T button name (\"OK\")")) -> (T button?=w391:bool)
        n174 = case shown="True" w391 {
          tunnel: w390 -> [w396 w397]
          tunnel: [w396 w403] -> w388
          tunnel: w389 -> [_ w398]
          frame False {
          }
          frame True {
            n175 = call-poly "Enqueue Message.vi"("error in (no error)"=w397, "Message"="Detener_Instrumento", "Message Queue"=w398) -> ("error out"=w399:errorcluster, "dup Message Queue"=w400:refnum<queue>)  [unwired: 7 in]
            n176 = call-poly "Enqueue Message.vi"("error in (no error)"=w399, "Message"="Exit", "Message Queue"=w400) -> ("error out"=w403:errorcluster)  [unwired: 7 in, 1 out]
          }
        }
      }
      frame "Error" {
        w411 = T8 1 items=["no dialog", "OK message", "continue or stop message", "OK message + warnings", "continue/stop + warnings"] ("type of dialog (OK msg:1)")
        n177 = Variant To Data(error in=w407, type=errorcluster {"status"=FALSE, "code"=0, "source"=""} ("error out"), Variant=w404) -> (data=w409:errorcluster, error out=w408:errorcluster)
        n178 = call <vilib>:"Simple Error Handler.vi"("type of dialog (OK msg:1)"=w411, "error in (no error)"=w409) -> ()  [unwired: 3 in, 5 out]
        n179 = call-poly "Enqueue Message.vi"("error in (no error)"=w408, "Message"="Exit", "Message Queue"=w406) -> ("error out"=w405:errorcluster)  [unwired: 7 in, 1 out]
      }
      frame Default {
        n180 = xnode "Error Ring"("parameter 0"=w415) -> ("error out"=w414:errorcluster)
      }
      frame "---------------Controles---------------" {
        n181 = xnode "Error Ring"("parameter 0"=w425) -> ("error out"=w424:errorcluster)
      }
    }
    n182 = call "Error Handler - Message Handling Loop.vi"("error in (no error)"=w89, "Message Queue"=w88) -> ("dup error in"=w87:errorcluster)  [unwired: 8 in, 1 out]
  }
  "Prueba05 out" <- w17
  n183 = call "Inst_CNT90.vi"("error in"=w5, "All Message Queues in"=w6, "Prueba31 in"=w7) -> ()  [unwired: 8 in, 1 out]
  n184 = call "Inst_DS360.vi"("error in"=w5, "All Message Queues in"=w6, "Prueba05 in"=w7) -> ()  [unwired: 8 in, 1 out]
  n185 = call "Inst_K2002.vi"("error in"=w5, "All Message Queues in"=w6, "Prueba31 in"=w7) -> ()  [unwired: 8 in, 1 out]
  n186 = Merge Errors(w20, w19) -> (→"error out":errorcluster)
